vi "get_component_type_name.vi"(8 "error in (no error)":errorcluster, 11 "GenericScanMode in":refnum<class "GenericImagingMode.lvclass">) -> (0 "error out":errorcluster, 2 "component type":string="ImagingMode", 3 "GenericScanMode out":refnum<class "GenericImagingMode.lvclass">)   [LabVIEW 2010, in "GenericImagingMode.lvclass"]
uses:
  GenericImagingMode.lvclass
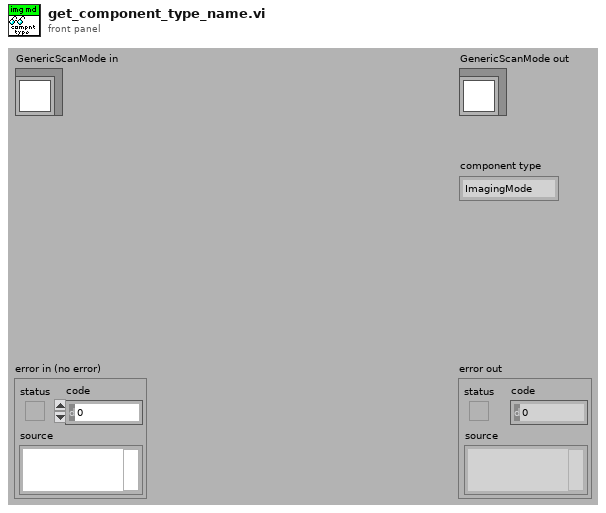
[diagram p1: front panel]
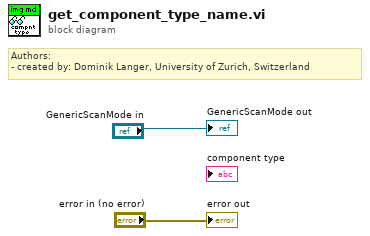
[diagram p0: block diagram]
diagram:
  # "Authors: \n- created by: Dominik Langer, University of Zurich, Switzerland"
  "error out" <- "error in (no error)"
  "GenericScanMode out" <- "GenericScanMode in"
